vi "lcr tune.vi"() -> ()   [LabVIEW 2018]
uses:
  <vilib>/DAQmx/write.llb/DAQmx Write (Analog DBL 1Chan 1Samp).vi
  2a3dda8a-b8aa-4613-8376-8d8c81e86704.vi
  <vilib>/DAQmx/read.llb/DAQmx Read (Analog DBL 1Chan 1Samp).vi
  <vilib>/Analysis/baseanly.llb/Mean (DBL).vi
  <vilib>/DAQmx/create/channels.llb/DAQmx Create Channel (AO-Voltage-Basic).vi
  <vilib>/DAQmx/miscellaneous.llb/DAQmx Fill In Error Info.vi
  <vilib>/DAQmx/create/channels.llb/DAQmx Create Channel (AI-Voltage-Basic).vi
  <vilib>/ptbypt/NI_PtbyPt.lvlib
  <vilib>/Analysis/NI_AALBase.lvlib
panel:
  out "threshold":dbl
  out "LCR Input Low":dbl=3.316831683168317
  out "LCR Input High":dbl=3.7623762376237626
  out "XY Graph 2":cluster{dbl[], dbl[]}(graph)={[0.0, 0.04950495049504951, 0.09900990099009901, 0.14851485148514854, 0.19801980198019803, 0.24752475247524752, 0.29702970297029707, 0.34653465346534656, 0.39603960396039606, 0.44554455445544555, 0.49504950495049505, 0.5445544554455446, 0.5940594059405941, 0.6435643564356436, 0.6930693069306931, 0.7425742574257426, 0.7920792079207921, 0.8415841584158417, 0.8910891089108911, 0.9405940594059407, 0.9900990099009901, 1.0396039603960396, 1.0891089108910892, 1.1386138613861387, 1.1881188118811883, 1.2376237623762376, 1.2871287128712872, 1.3366336633663367, 1.3861386138613863, 1.4356435643564358, 1.4851485148514851, 1.5346534653465347, 1.5841584158415842, 1.6336633663366338, 1.6831683168316833, 1.7326732673267327, 1.7821782178217822, 1.8316831683168318, 1.8811881188118813, 1.9306930693069309, 1.9801980198019802, 2.0297029702970297, 2.0792079207920793, 2.128712871287129, 2.1782178217821784, 2.227722772277228, 2.2772277227722775, 2.326732673267327, 2.3762376237623766, 2.4257425742574257, 2.4752475247524752, 2.5247524752475248, 2.5742574257425743, 2.623762376237624, 2.6732673267326734, 2.722772277227723, 2.7722772277227725, 2.821782178217822, 2.8712871287128716, 2.9207920792079207, 2.9702970297029703, 3.01980198019802, 3.0693069306930694, 3.118811881188119, 3.1683168316831685, 3.217821782178218, 3.2673267326732676, 3.316831683168317, 3.3663366336633667, 3.415841584158416, 3.4653465346534653, 3.514851485148515, 3.5643564356435644, 3.613861386138614, 3.6633663366336635, 3.712871287128713, 3.7623762376237626, 3.811881188118812, 3.8613861386138617, 3.9108910891089113, 3.9603960396039604, 4.00990099009901, 4.0594059405940595, 4.108910891089109, 4.158415841584159, 4.207920792079208, 4.257425742574258, 4.306930693069307, 4.356435643564357, 4.405940594059406, 4.455445544554456, 4.504950495049505, 4.554455445544555, 4.6039603960396045, 4.653465346534654, 4.702970297029704, 4.752475247524753, 4.801980198019802, 4.851485148514851, 4.900990099009901, 4.9504950495049505, 5.0], [3.6269698987299557, 3.6364573449364106, 3.6329899671345474, 3.6282543529705342, 3.629159309363951, 3.6287473758170243, 3.6300350736155056, 3.629924792216151, 3.6336451685832807, 3.63122870790565, 3.6250464609928272, 3.6300902143756275, 3.637209853485964, 3.6333467600149016, 3.630025342964688, 3.6329121214483715, 3.6278326887176044, 3.6270445008971244, 3.6230613953263267, 3.630712980049897, 3.6313000664504536, 3.6289971308177837, 3.6302329315360238, 3.6329153650017383, 3.6294609615211413, 3.63600000136827, 3.627411024462163, 3.6284100444363565, 3.6275861772915365, 3.6304729557761015, 3.629473935783759, 3.63204933151817, 3.6254162280427176, 3.627398050221512, 3.6295193457817647, 3.6331878249951624, 3.6319941907248854, 3.6278034965744808, 3.6220396703232898, 3.6262952359408596, 3.6273688580229018, 3.6348777256768994, 3.6264476837299795, 3.633719770708133, 3.6360843342001994, 3.6295290764943395, 3.6302459057692227, 3.6275504979969018, 3.6291366044222984, 3.632672097159256, 3.6235057645788302, 3.6296361143819986, 3.6328342757014656, 3.6316990257371065, 3.62449829739106, 3.629097681502316, 3.624031223133673, 3.6252702673373305, 3.6278229579737187, 3.6336192199758655, 3.6273623709287937, 3.621828838189813, 3.631844986473933, 3.625150255217819, 3.625172960190463, 3.6291917451084803, 3.6294479872235597, 3.619243711878944, 3.6345630992469626, 3.6295615122275064, 3.6293896029595634, 3.6309984143274994, 3.6328083271841956, 3.6245664123692127, 3.6280954180164486, 3.627754843002688, 3.6386662170654303, 3.62156935249656, 3.6349231357495135, 3.637310404233228, 3.6250724094892646, 3.6337684242639474, 3.638114809914663, 3.625224857360931, 3.6308427229410554, 3.637796939897928, 3.6351177500173657, 3.6332105299869375, 3.632360714266952, 3.635607529201048, 3.6308200179121477, 3.634835559237383, 3.6350820706466345, 3.6253027030898712, 3.633823564980328, 3.623252765981493, 3.6300156121881697, 3.6215855703379147, 3.6359124249670454, 3.630398353613972, 3.6265287730372937, 3.6269212451486847]}
  in  "laser tune voltage":dbl=3.79 min=0.0 max=4.0 step=0.01
  out "Current Voltage":dbl=5.0
  # "This VI sweeps the LCR driving voltage.   LCR slow axis should be aligned to roughly 45 degrees from the \ntransmission axis of the linear plarizer.  The max and min of graph represent citical values such as 1/4 wave,\n3/4 wave, etc.  The corresponding Voltages are then used fine tune the alignemnt and to make polarization\nmeasurements."
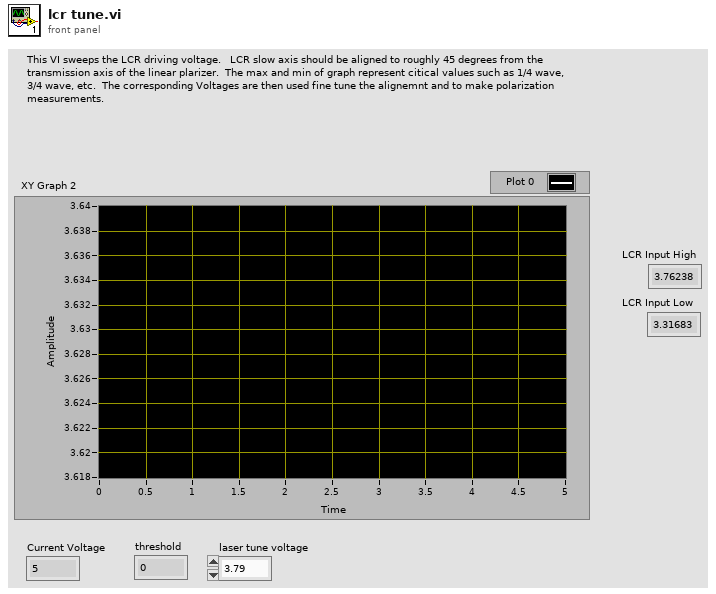
[diagram p1: front panel]
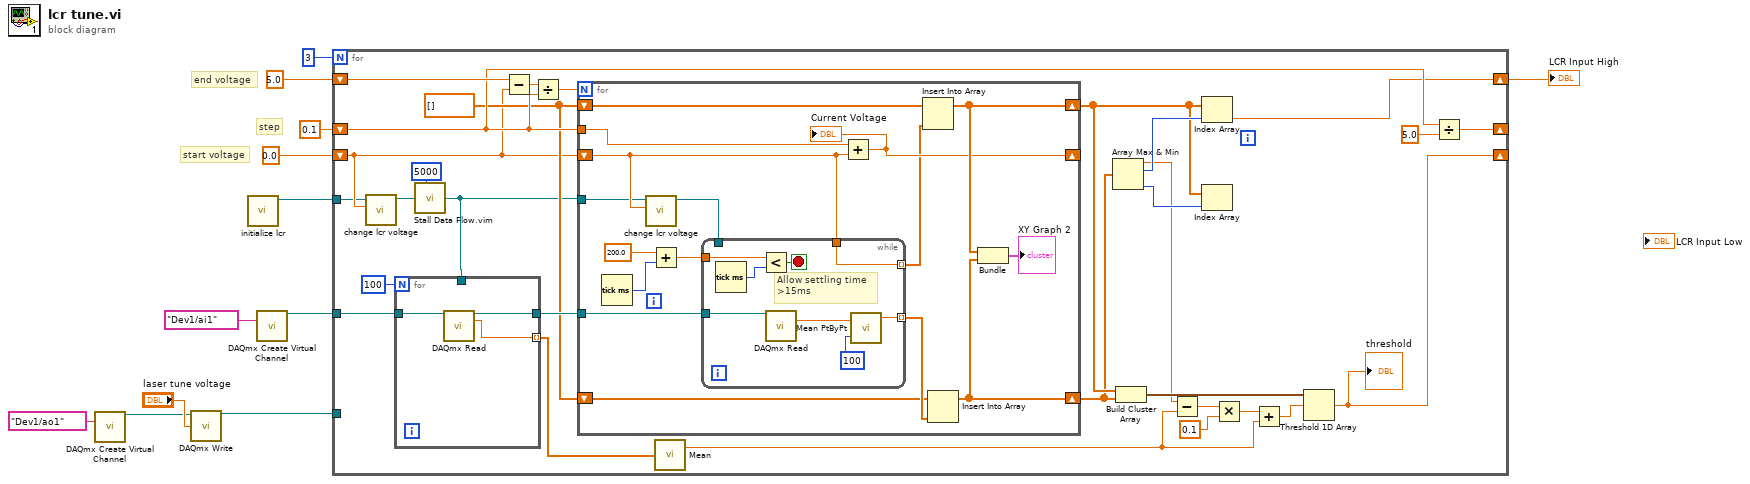
[diagram p0: block diagram]
diagram:
  # "step"
  # "start voltage"
  # "end voltage"
  n1 = call-poly <vilib>:"DAQmx Create Virtual Channel.vi"("physical channels"=tag "Dev1/ao1") -> ("task out"=w9:refnum<k21>)  [unwired: 13 in, 1 out]
  n2 = call-poly <vilib>:"DAQmx Write.vi"("task/channels in"=w9, "data"="laser tune voltage") -> ("task out"=w4:refnum<k21>)  [unwired: 11 in, 2 out]
  n3 = call "initialize lcr.vi"() -> ("lcr out"=w2:refnum<visa-resource-name>)  [unwired: 11 in]
  n4 = call-poly <vilib>:"DAQmx Create Virtual Channel.vi"("physical channels"=tag "Dev1/ai1") -> ("task out"=w5:refnum<k21>)  [unwired: 13 in, 1 out]
  n5 = for {
    N: 3 -> [_]
    shift-right: [w27] -> _
    shift-left: 0.1 ("step size") -> [w26]
    shift-right: [w28] -> _
    shift-left: 0.0 ("Start Voltage") -> [w17]
    shift-right: [w13] -> w1
    shift-left: 5.0 ("End Voltage") -> [w30]
    tunnel: w5 -> [w20]
    tunnel: w4 -> [_]
    tunnel: w2 -> [w16]
    w19 = dbl[] []
    n6 = call "change lcr voltage.vi"("voltage"=w17, "lcr in"=w16) -> ("lcr out"=w18:refnum<visa-resource-name>)  [unwired: 9 in]
    n7 = call "Stall Data Flow.vim"("value in"=w18, "milliseconds to wait"=u32 5000) -> ("value out"=w14:refnum<visa-resource-name>)  [unwired: 1 out]
    n8 = for {
      N: 100 -> [_]
      tunnel: [w44] -> w22
      tunnel: [w43] -> w21 mode=indexing
      tunnel: w20 -> [w42]
      tunnel: w14 -> [_]
      n9 = call-poly <vilib>:"DAQmx Read.vi"("task/channels in"=w42) -> ("task out"=w44:refnum<k21>, "data"=w43:dbl)  [unwired: 12 in, 1 out]
    }
    n10 = Subtract(x=w30, y=w17) -> (x-y=w29:dbl)
    n11 = Divide(x=w29, y=w26) -> (x/y=w31:dbl)
    n12 = for {
      N: w31 -> [_]
      tunnel: w14 -> [w46]
      shift-right: [w49] -> _
      shift-left: w17 -> [w47]
      tunnel: w26 -> [w53]
      tunnel: w22 -> [w60]
      shift-right: [w51] -> w33
      shift-left: w19 -> [w54]
      shift-right: [w52] -> w34
      shift-left: w19 -> [w55]
      n13 = Tick Count (ms)() -> (millisecond timer value=w59:u32)
      n14 = call "change lcr voltage.vi"("voltage"=w47, "lcr in"=w46) -> ("lcr out"=w45:refnum<visa-resource-name>)  [unwired: 9 in]
      n15 = Add(x=200.0 ("Step length (ms)"), y=w59) -> (x+y=w57:dbl)
      n16 = while {
        tunnel: w60 -> [w68]
        tunnel: w57 -> [w67]
        tunnel: [w62] -> w56 mode=indexing
        tunnel: w47 -> [w61]
        tunnel: [w61] -> w48 mode=indexing
        tunnel: w45 -> [_]
        stop <- w65 stop-if-true
        # "Allow settling time\n>15ms"
        n17 = Tick Count (ms)() -> (millisecond timer value=w66:u32)
        n18 = Less?(x=w67, y=w66) -> (x < y?=w65:bool)
        n19 = call-poly <vilib>:"DAQmx Read.vi"("task/channels in"=w68) -> ("data"=w64:dbl)  [unwired: 12 in, 2 out]
        n20 = call <vilib>:"Mean PtByPt.vi"("x"=w64, "sample length"=100) -> ("mean"=w62:dbl)  [unwired: 2 in, 1 out]
      }
      n21 = Add(x=w53, y=w47) -> (x+y=w49:dbl)
      "Current Voltage" <- w49
      n22 = Insert Into Array(array=w55, new element=w48) -> (w52:dbl[])  [unwired: 1 in]
      n23 = Insert Into Array(array=w54, new element=w56) -> (w51:dbl[])  [unwired: 1 in]
      n24 = Bundle(w52, w51) -> (→"XY Graph 2":cluster{dbl[], dbl[]})  [unwired: 1 in]
    }
    n25 = call-poly <vilib>:"Mean.vi"("X"=w21) -> ("mean"=w24:dbl)  [unwired: 1 out]
    n26 = Array Max & Min(array=w33) -> (max value=w32:dbl, max index (indices)=w37:i32, min index (indices)=w36:i32)  [unwired: 1 out]
    n27 = Build Cluster Array(w34, w33) -> (w38:cluster{dbl, dbl}[])
    n28 = Subtract(x=w32, y=w24) -> (x-y=w39:dbl)
    n29 = Index Array(array=w34, index=w37) -> (element=w13:dbl)
    n30 = Index Array(array=w34, index=w36) -> ()  [unwired: 1 out]
    n31 = Multiply(x=w39, y=0.1) -> (x*y=w40:dbl)
    n32 = Add(x=w40, y=w24) -> (x+y=w41:dbl)
    n33 = Threshold 1D Array(2:w41, 3:w38) -> (0:w28:dbl)  [unwired: 1 in]
    "threshold" <- w28
    n34 = Divide(x=w26, y=5.0) -> (x/y=w27:dbl)
  }
  "LCR Input High" <- w1
